vi "Configure Measurement.vi"(0 "VISA resource name":refnum<visa-resource-name>, 1 "Ref Level Calculate Method (0: Auto Select)":i32(ring) items=["Auto Select", "Histogram", "Min/Max"], 2 "Gating (0: Screen)":u16(ring) items=["Screen", "Between Cursors", "Off"], 5 "High Ref (90%)":dbl=90.0, 7 "Mid Ref (50%)":dbl=50.0, 9 "Low Ref (10%)":dbl=10.0, 11 "error in (no error)":errorcluster, 12 "Second Source Mid Ref (50%)":dbl=50.0) -> (4 "VISA resource name out":refnum<visa-resource-name>, 15 "error out":errorcluster)   [LabVIEW 2009, in "Tektronix DPO MSO 2000 4000 Series.lvlib"]
doc: "Configures the reference levels and method an oscilloscope uses to calculate the measurement reference levels. This VI also controls the gating method for measurements."
uses:
  <instrlib>/Tektronix DPO MSO 2000 4000 Series/Tektronix DPO MSO 2000 4000 Series.lvlib
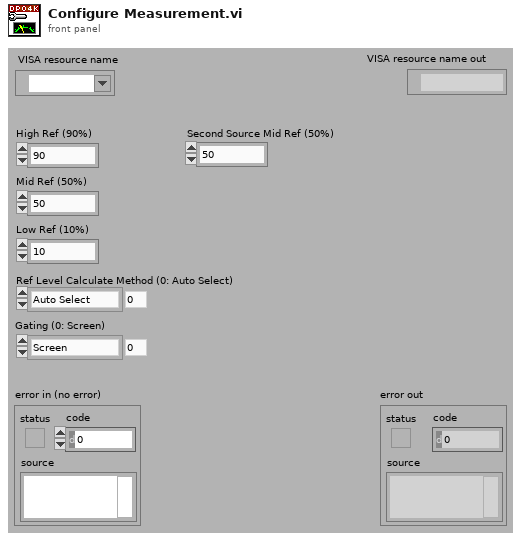
[diagram p1: front panel]
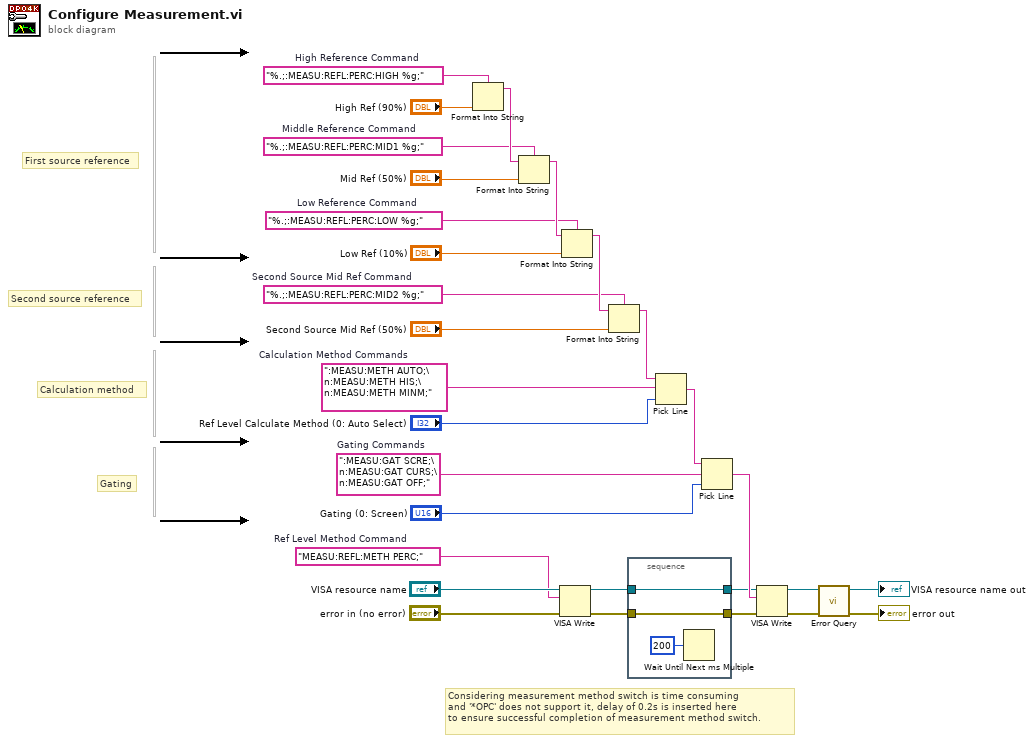
[diagram p0: block diagram]
diagram:
  w1 = "MEASU:REFL:METH PERC;"  # Ref Level Method Command
  w15 = ":MEASU:GAT SCRE;\n:MEASU:GAT CURS;\n:MEASU:GAT OFF;"  # Gating Commands
  w19 = ":MEASU:METH AUTO;\n:MEASU:METH HIS;\n:MEASU:METH MINM;"  # Calculation Method Commands
  w8 = "%.;:MEASU:REFL:PERC:MID2 %g;"  # Second Source Mid Ref Command
  w22 = "%.;:MEASU:REFL:PERC:LOW %g;"  # Low Reference Command
  w25 = "%.;:MEASU:REFL:PERC:MID1 %g;"  # Middle Reference Command
  w28 = "%.;:MEASU:REFL:PERC:HIGH %g;"  # High Reference Command
  # "Considering measurement method switch is time consuming\nand '*OPC' does not support it, delay of 0.2s is inserted here \nto ensure successful completion of measurement method switch."
  # "Gating"
  # "Calculation method"
  # "Second source reference"
  # "First source reference"
  n1 = Format Into String(format string=w28, "High Ref (90%)") -> (resulting string=w27:string)  [unwired: 2 in, 1 out]
  n2 = Format Into String(format string=w25, initial string=w27, "Mid Ref (50%)") -> (resulting string=w24:string)  [unwired: 1 in, 1 out]
  n3 = VISA Write(VISA resource name="VISA resource name", write buffer=w1, error in (no error)="error in (no error)") -> (VISA resource name out=w7:refnum<visa-resource-name>, error out=w6:errorcluster)  [unwired: 1 out]
  n4 = Format Into String(format string=w22, initial string=w24, "Low Ref (10%)") -> (resulting string=w21:string)  [unwired: 1 in, 1 out]
  n5 = Format Into String(format string=w8, initial string=w21, "Second Source Mid Ref (50%)") -> (resulting string=w17:string)  [unwired: 1 in, 1 out]
  n6 = stacked-sequence {
    tunnel: w7 -> [w31]
    tunnel: [w31] -> w3
    tunnel: w6 -> [w30]
    tunnel: [w30] -> w2
    frame #0 {
      n7 = Wait Until Next ms Multiple(millisecond multiple=u32 200) -> ()  [unwired: 1 out]
    }
  }
  n8 = Pick Line(string ("")=w17, multi-line string=w19, line index="Ref Level Calculate Method (0: Auto Select)") -> (output string=w16:string)
  n9 = Pick Line(string ("")=w16, multi-line string=w15, line index="Gating (0: Screen)") -> (output string=w13:string)
  n10 = VISA Write(VISA resource name=w3, write buffer=w13, error in (no error)=w2) -> (VISA resource name out=w12:refnum<visa-resource-name>, error out=w11:errorcluster)  [unwired: 1 out]
  n11 = call <instrlib>:"Error Query.vi"("error in (no error)"=w11, "VISA resource name"=w12) -> ("error out"=→"error out":errorcluster, "VISA resource name out"=→"VISA resource name out":refnum<visa-resource-name>)  [unwired: 6 in, 2 out]
